vi "Meacurrent.vi"(10 "测试类型":u16(ring) items=["DCV", "ACV", "DCI", "ACI", "OHM", "RST", "CAP", "FRQ", "AUTO"], 11 "VISA资源名称":refnum<visa-resource-name>="COM1") -> (0 "错误输出":errorcluster, 2 "数值":dbl format="%#_3g")   [LabVIEW 2013]
uses:
  C:/Program Files/National Instruments/LabVIEW 2013/examples/Instrument IO/Serial/support/Serial - Settings.ctl
  <vilib>/Instr/_visa.llb/VISA Configure Serial Port (Instr).vi
panel:
  out "响应":string
  in  "串口设置":T1={"波特率"=9600, "数据比特"=8, "奇偶"=enum."None", "停止位"=10, "流控制"=0} {"流控制" items=["无"=0, "XON/XOFF"=1, "RTS/CTS"=2, "DTR/DSR"=4]; "停止位" items=["1.0"=10, "1.5"=15, "2.0"=20]; "数据比特" min=5 max=8 step=1; "波特率" items=["75"=75, "110"=110, "134"=134, "150"=150, "300"=300, "600"=600, "1200"=1200, "1800"=1800, "2400"=2400, "4800"=4800, "7200"=7200, "9600"=9600, "14400"=14400, "19200"=19200, "28800"=28800, "38400"=38400, "56000"=56000, "57600"=57600, "115200"=115200, "128000"=128000, "230400"=230400]}
  in  "读取前延时(ms)":u32=600
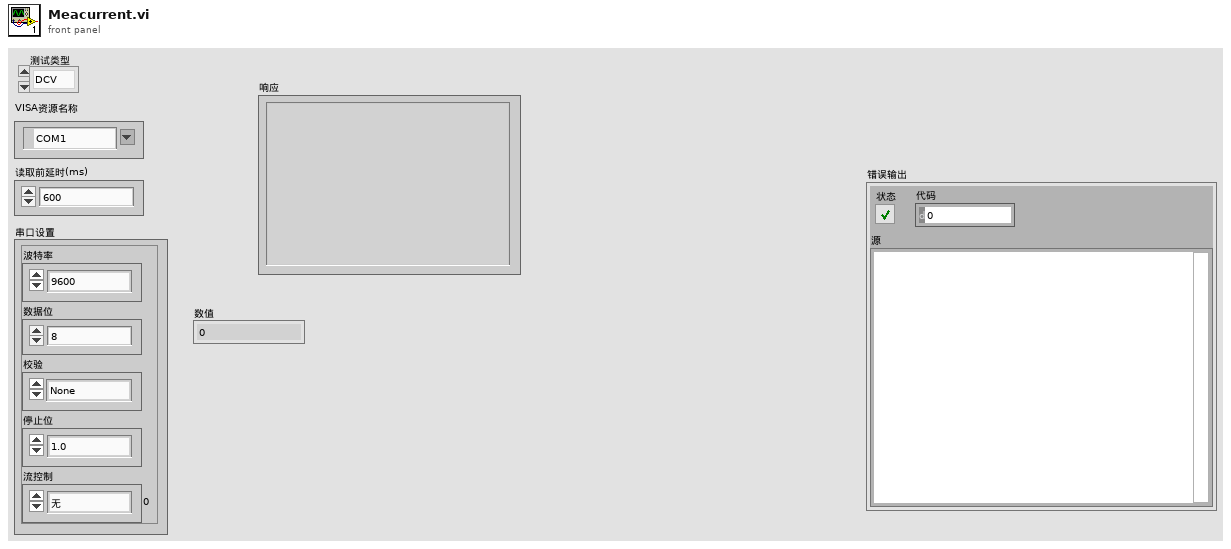
[diagram p1: front panel]
types:
  T1 = typedef "Serial - Settings.ctl" = cluster{"波特率":u32, "数据比特":u16, "奇偶":enum16{"None", "Odd", "Even", "Mark", "Space"}, "停止位":u16, "流控制":u16}
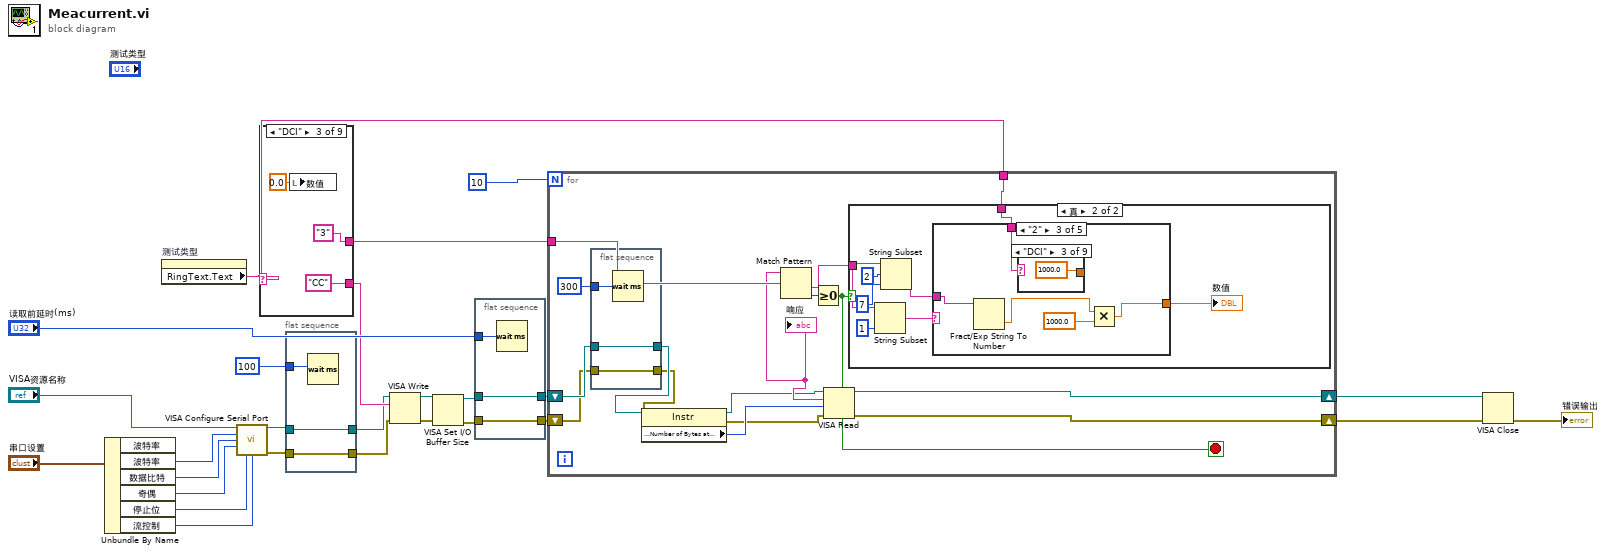
[diagram p0: block diagram]
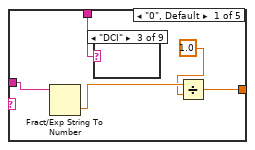
[diagram p3: hidden frame]
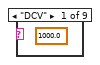
[diagram p4: hidden frame]
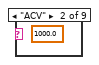
[diagram p5: hidden frame]
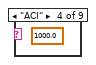
[diagram p6: hidden frame]
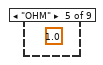
[diagram p7: hidden frame]
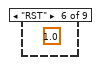
[diagram p8: hidden frame]
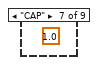
[diagram p9: hidden frame]
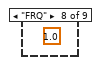
[diagram p10: hidden frame]
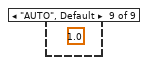
[diagram p11: hidden frame]
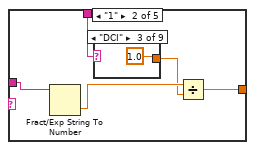
[diagram p12: hidden frame]
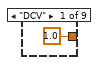
[diagram p13: hidden frame]
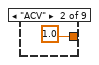
[diagram p14: hidden frame]
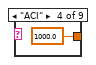
[diagram p15: hidden frame]
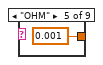
[diagram p16: hidden frame]
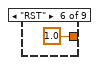
[diagram p17: hidden frame]
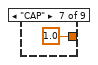
[diagram p18: hidden frame]
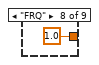
[diagram p19: hidden frame]
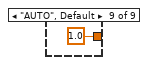
[diagram p20: hidden frame]
diagram:
  n1 = Unbundle By Name("串口设置") -> ("波特率"=w19:u32, "数据比特"=w18:u16, "奇偶"=w17:enum16{"None", "Odd", "Even", "Mark", "Space"}, "停止位"=w16:u16, "流控制"=w15:u16)  [unwired: 1 out]
  n2 = property on="测试类型" class="Ring (严格)"() -> ("RingText.Text"=w12:string)  [unwired: 2 in, 2 out]
  n3 = call-poly "VISA Configure Serial Port"("VISA resource name"="VISA资源名称", "baud rate (9600)"=w19, "data bits (8)"=w18, "parity (0:none)"=w17, "stop bits (10: 1 bit)"=w16, "flow control (0:none)"=w15) -> ("VISA resource name out"=w9:refnum<visa-resource-name>, "error out"=w8:errorcluster)  [unwired: 3 in, 5 out]
  n4 = case shown="\"DCI\"" w12 {
    tunnel: ["AA" ("Command") "BB" ("Command") "CC" ("Command") "DD" ("Command") "EE" ("Command") "FF" ("Command") "GG" ("Command") "HH" ("Command") "MM" ("Command")] -> w14
    tunnel: ["0" ("Command") "1" ("Command") "3" ("Command") "4" ("Command") "6" ("Command") "F" ("Command") "7" ("Command") "8" ("Command") "M" ("Command")] -> w13
    frame "DCV" {
    }
    frame "ACV" {
    }
    frame "DCI" {
      n5 = local write "数值"(0.0 ("数值")) -> ()
    }
    frame "ACI" {
    }
    frame "OHM" {
    }
    frame "RST" {
    }
    frame "CAP" {
    }
    frame "FRQ" {
    }
    frame "AUTO", Default {
    }
  }
  n6 = flat-sequence {
    tunnel: w8 -> [w48]
    tunnel: [w48] -> w7
    tunnel: [w47] -> w6
    tunnel: w9 -> [w47]
    tunnel: u32 100 ("读取前延时(ms)") -> [w46]
    frame #0 {
      n7 = Wait (ms)(milliseconds to wait=w46) -> ()  [unwired: 1 out]
    }
  }
  n8 = VISA Write(VISA resource name=w6, write buffer=w14, error in (no error)=w7) -> (VISA resource name out=w3:refnum<visa-resource-name>, error out=w4:errorcluster)  [unwired: 1 out]
  n9 = VISA Set I/O Buffer Size(VISA resource name=w3, error in (no error)=w4) -> (VISA resource name out=w2:refnum<visa-resource-name>, error out=w1:errorcluster)  [unwired: 2 in]
  n10 = flat-sequence {
    tunnel: w1 -> [w49]
    tunnel: [w49] -> w23
    tunnel: [w50] -> w22
    tunnel: "读取前延时(ms)" -> [w51]
    tunnel: w2 -> [w50]
    frame #0 {
      n11 = Wait (ms)(milliseconds to wait=w51) -> ()  [unwired: 1 out]
    }
  }
  n12 = for {
    N: 10 -> [_]
    tunnel: w13 -> [w64]
    tunnel: w12 -> [w60]
    shift-right: [w66] -> w24
    shift-left: w22 -> [w59]
    shift-right: [w67] -> w25
    shift-left: w23 -> [w57]
    stop <- w54 stop-if-true
    n13 = flat-sequence {
      tunnel: w57 -> [w69]
      tunnel: [w69] -> w56
      tunnel: w59 -> [w68]
      tunnel: [w68] -> w58
      tunnel: u32 300 ("读取前延时(ms)") -> [w70]
      frame #0 {
        n14 = Wait (ms)(milliseconds to wait=w70) -> ()  [unwired: 1 out]
      }
    }
    n15 = property class="Instr"(reference=w58, error in=w56) -> (reference out=w53:refnum<visa-resource-name>, error out=w52:errorcluster, "Serial Settings:Number of Bytes at Serial Port"=w65:u32)
    n16 = VISA Read(VISA resource name=w53, byte count=w65, error in (no error)=w52) -> (VISA resource name out=w66:refnum<visa-resource-name>, read buffer=w61:string, error out=w67:errorcluster)  [unwired: 1 out]
    "响应" <- w61
    n17 = Match Pattern(string=w61, regular expression=w64) -> (after substring=w62:string, offset past match=w63:i32)  [unwired: 1 in, 2 out]
    n18 = Greater Or Equal To 0?(x=w63) -> (x >= 0?=w54:bool)
    n19 = case shown="真" w54 {
      tunnel: w62 -> [_ w76]
      tunnel: w60 -> [_ w72]
      frame False {
      }
      frame True {
        n20 = String Subset(string=w76, length (rest)=1 ("长度（剩余）")) -> (substring=w77:string)  [unwired: 1 in]
        n21 = String Subset(string=w76, offset (0)=2 ("偏移量(0)"), length (rest)=7 ("长度（剩余）")) -> (substring=w73:string)
        n22 = case shown="\"2\"" w77 {
          tunnel: w73 -> [w83 w88 w102 w116 w130]
          tunnel: w72 -> [w82 w87 w101 w115 w129]
          tunnel: [w80 w84 w98 w112 w126] -> w71
          frame "0", Default {
            n23 = Fract/Exp String To Number(string=w83) -> (number=w81:dbl)  [unwired: 3 in, 1 out]
            n24 = case shown="\"DCI\"" w82 {
              frame "DCV" {
                (unwired) 1000.0
              }
              frame "ACV" {
                (unwired) 1000.0
              }
              frame "DCI" {
              }
              frame "ACI" {
                (unwired) 1000.0
              }
              frame "OHM" {
                (unwired) 1.0
              }
              frame "RST" {
                (unwired) 1.0
              }
              frame "CAP" {
                (unwired) 1.0
              }
              frame "FRQ" {
                (unwired) 1.0
              }
              frame "AUTO", Default {
                (unwired) 1.0
              }
            }
            n25 = Divide(x=w81, y=1.0 ("数字")) -> (x/y=w80:dbl)
          }
          frame "1" {
            n26 = Fract/Exp String To Number(string=w88) -> (number=w86:dbl)  [unwired: 3 in, 1 out]
            n27 = case shown="\"DCI\"" w87 {
              tunnel: [1.0 1.0 1.0 1000.0 0.001 1.0 1.0 1.0 1.0] -> w85
              frame "DCV" {
              }
              frame "ACV" {
              }
              frame "DCI" {
              }
              frame "ACI" {
              }
              frame "OHM" {
              }
              frame "RST" {
              }
              frame "CAP" {
              }
              frame "FRQ" {
              }
              frame "AUTO", Default {
              }
            }
            n28 = Divide(x=w86, y=w85) -> (x/y=w84:dbl)
          }
          frame "2" {
            n29 = Fract/Exp String To Number(string=w102) -> (number=w100:dbl)  [unwired: 3 in, 1 out]
            n30 = case shown="\"DCI\"" w101 {
              tunnel: [1.0 1.0 1000.0 1000.0 0.001 1.0 1.0 1.0 1.0] -> _
              frame "DCV" {
              }
              frame "ACV" {
              }
              frame "DCI" {
              }
              frame "ACI" {
              }
              frame "OHM" {
              }
              frame "RST" {
              }
              frame "CAP" {
              }
              frame "FRQ" {
              }
              frame "AUTO", Default {
              }
            }
            n31 = Multiply(x=w100, y=1000.0) -> (x*y=w98:dbl)
          }
          frame "3" {
            n32 = Fract/Exp String To Number(string=w116) -> (number=w114:dbl)  [unwired: 3 in, 1 out]
            n33 = case shown="\"DCI\"" w115 {
              tunnel: [1.0 1.0 1000.0 1000.0 0.001 1.0 1.0 1.0 1.0] -> w113
              frame "DCV" {
              }
              frame "ACV" {
              }
              frame "DCI" {
              }
              frame "ACI" {
              }
              frame "OHM" {
              }
              frame "RST" {
              }
              frame "CAP" {
              }
              frame "FRQ" {
              }
              frame "AUTO", Default {
              }
            }
            n34 = Divide(x=w114, y=w113) -> (x/y=w112:dbl)
          }
          frame "4" {
            n35 = Fract/Exp String To Number(string=w130) -> (number=w128:dbl)  [unwired: 3 in, 1 out]
            n36 = case shown="\"DCI\"" w129 {
              tunnel: [1.0 1.0 1000.0 1000.0 1e-06 1.0 1.0 1.0 1.0] -> w127
              frame "DCV" {
              }
              frame "ACV" {
              }
              frame "DCI" {
              }
              frame "ACI" {
              }
              frame "OHM" {
              }
              frame "RST" {
              }
              frame "CAP" {
              }
              frame "FRQ" {
              }
              frame "AUTO", Default {
              }
            }
            n37 = Divide(x=w128, y=w127) -> (x/y=w126:dbl)
          }
        }
        "数值" <- w71
      }
    }
  }
  n38 = VISA Close(VISA resource name=w24, error in (no error)=w25) -> (error out=→"错误输出":errorcluster)
